vi "TagMetadataToImage.vi"(8 "error in (no error)":errorcluster, 10 "Image In":T1, 11 "Stage_MadCityLabMicro in":refnum<class "Stage_MadCityLabMicro.lvclass">) -> (0 "error out":errorcluster, 2 "Image Out":T1, 3 "Stage_MadCityLabMicro out":refnum<class "Stage_MadCityLabMicro.lvclass">)   [LabVIEW 2020, in "Stage_MadCityLabMicro.lvlib" / "Stage_MadCityLabMicro.lvclass"]
uses:
  Stage_MadCityLabMicro.lvclass
  <vilib>/vision/Image Controls.llb/IMAQ Image.ctl
  Stage_MadCityLabMicro.lvclass/Stage_MadCityLabMicro.ctl
  Hardware Abstraction Layer/Component/Stage/Stage/Stage.lvclass
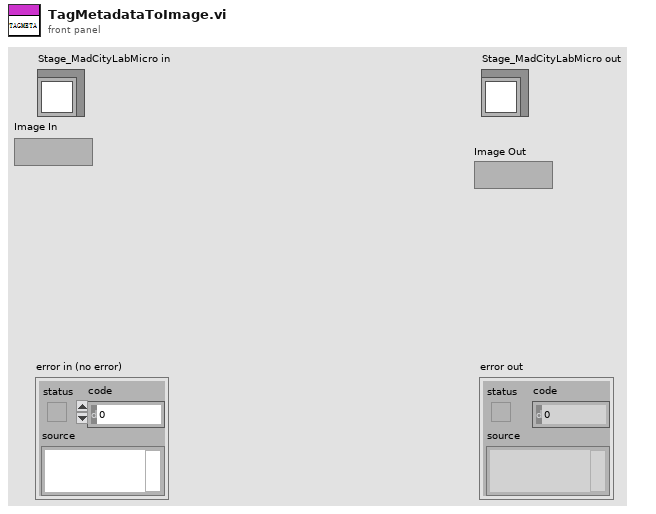
[diagram p1: front panel]
types:
  T1 = typedef "IMAQ Image.ctl" = refnum<image>
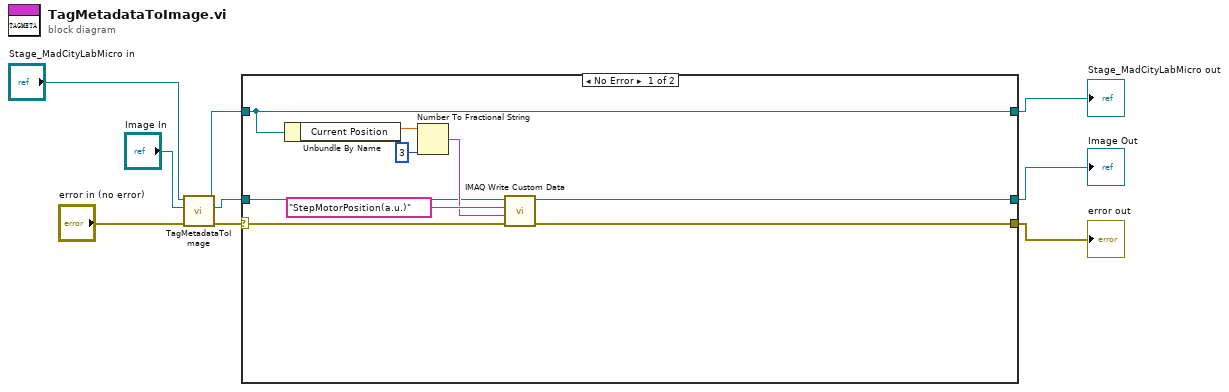
[diagram p0: block diagram]
diagram:
  n1 = call-parent "TagMetadataToImage.vi"("error in (no error)"="error in (no error)", "Image In"="Image In", "Device in"="Stage_MadCityLabMicro in") -> ("error out"=w6:errorcluster, "Image Out"=w5:T1, "Device out"=w4:refnum<class "Stage_MadCityLabMicro.lvclass">)  [unwired: 6 in]
  n2 = case shown="No Error" w6 {
    selector: w6 -> [w16 w21]
    tunnel: [w15 w21] -> w1
    tunnel: w5 -> [w12 w20]
    tunnel: [w11 w20] -> w2
    tunnel: [w18 w19] -> w3
    tunnel: w4 -> [w18 w19]
    frame No Error {
      n3 = Unbundle By Name(w18) -> ("Current Position"=w17:dbl)
      n4 = Number To Fractional String(number=w17, precision (6)=i16 3 ("width (-)")) -> (F-format string=w13:string)  [unwired: 2 in]
      n5 = call "IMAQ Write Custom Data"("error in (no error)"=w16, "Custom Data In"=w13, "Key"="StepMotorPosition(a.u.)", "Image"=w12) -> ("error out"=w15:errorcluster, "Image Out"=w11:T1)  [unwired: 6 in]
    }
    frame Error {
    }
  }
  "error out" <- w1
  "Stage_MadCityLabMicro out" <- w3
  "Image Out" <- w2
